vi "Test CAN write.vi"() -> ()   [LabVIEW 2023, in "PCAN API.lvlib"]
uses:
  PCAN API.lvlib
panel:
  in  "stop":bool
  out "MessageBuffer out":T1
  in  "MessageBuffer":T2(array[cluster])=[{"ID"=225, "MSGTYPE"=0, "LEN"=8, "DATA[0]"=0, "DATA[1]"=6, "DATA[2]"=0, "DATA[3]"=6, "DATA[4]"=0, "DATA[5]"=6, "DATA[6]"=0, "DATA[7]"=0}, {"ID"=225, "MSGTYPE"=0, "LEN"=8, "DATA[0]"=0, "DATA[1]"=0, "DATA[2]"=6, "DATA[3]"=2, "DATA[4]"=0, "DATA[5]"=5, "DATA[6]"=0, "DATA[7]"=0}, {"ID"=225, "MSGTYPE"=0, "LEN"=8, "DATA[0]"=8, "DATA[1]"=0, "DATA[2]"=0, "DATA[3]"=7, "DATA[4]"=0, "DATA[5]"=0, "DATA[6]"=0, "DATA[7]"=0}, {"ID"=225, "MSGTYPE"=0, "LEN"=8, "DATA[0]"=0, "DATA[1]"=0, "DATA[2]"=5, "DATA[3]"=0, "DATA[4]"=0, "DATA[5]"=0, "DATA[6]"=6, "DATA[7]"=0}, {"ID"=225, "MSGTYPE"=0, "LEN"=8, "DATA[0]"=0, "DATA[1]"=0, "DATA[2]"=7, "DATA[3]"=8, "DATA[4]"=8, "DATA[5]"=0, "DATA[6]"=0, "DATA[7]"=0}, {"ID"=225, "MSGTYPE"=0, "LEN"=8, "DATA[0]"=0, "DATA[1]"=3, "DATA[2]"=4, "DATA[3]"=6, "DATA[4]"=0, "DATA[5]"=0, "DATA[6]"=0, "DATA[7]"=0}, {"ID"=225, "MSGTYPE"=0, "LEN"=8, "DATA[0]"=1, "DATA[1]"=1, "DATA[2]"=1, "DATA[3]"=1, "DATA[4]"=0, "DATA[5]"=0, "DATA[6]"=0, "DATA[7]"=0}] {"ID" format="%.0x"}
  out "error out 2":errorcluster
  out "error out":errorcluster
  in  "error in":errorcluster
  in  "Channel":u16=81 format="%x"
  in  "IOPort":u32 format="%x"
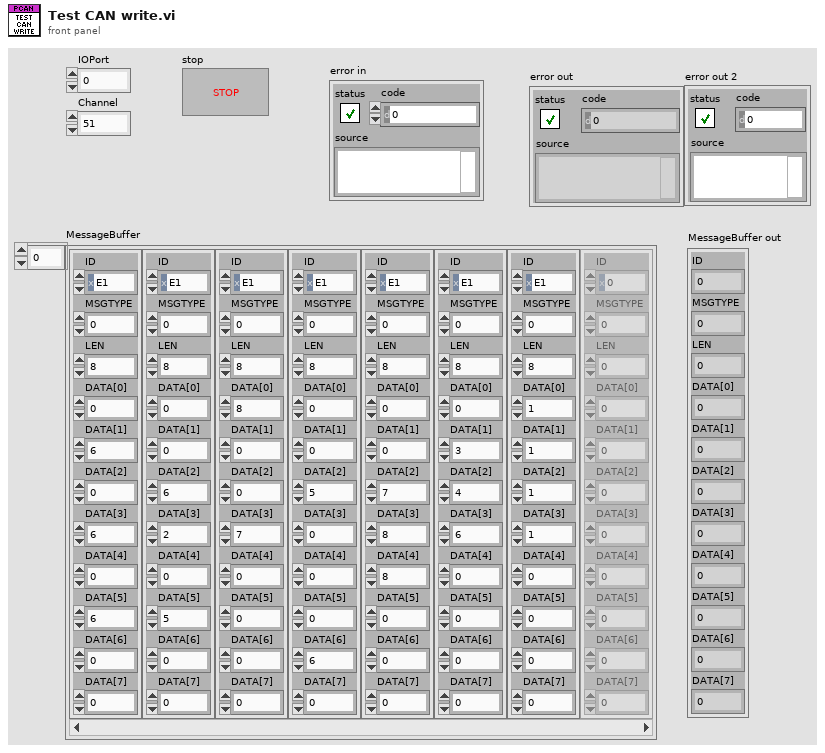
[diagram p1: front panel]
types:
  T1 = cluster{"ID":u32, "MSGTYPE":u8, "LEN":u8, "DATA[0]":u8, "DATA[1]":u8, "DATA[2]":u8, "DATA[3]":u8, "DATA[4]":u8, "DATA[5]":u8, "DATA[6]":u8, "DATA[7]":u8}
  T2 = cluster{"ID":u32, "MSGTYPE":u8, "LEN":u8, "DATA[0]":u8, "DATA[1]":u8, "DATA[2]":u8, "DATA[3]":u8, "DATA[4]":u8, "DATA[5]":u8, "DATA[6]":u8, "DATA[7]":u8}[]
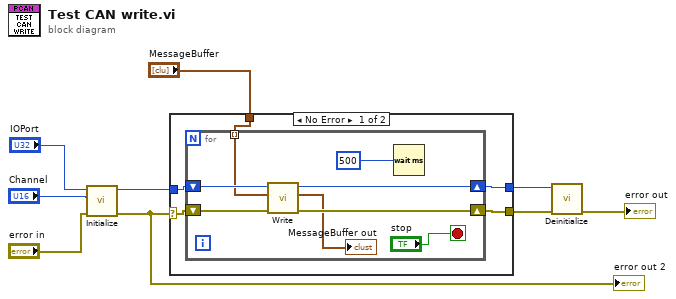
[diagram p0: block diagram]
diagram:
  n1 = call "Initialize.vi"("error in"="error in", "Channel"="Channel", "IOPort"="IOPort") -> ("error out"=w2:errorcluster, "Channel"=w6:u16)  [unwired: 6 in, 1 out]
  "error out 2" <- w2
  n2 = case shown="No Error" w2 {
    selector: w2 -> [w14 w23]
    tunnel: [w13 w23] -> w4
    tunnel: w6 -> [w12 w24]
    tunnel: [w11 w24] -> w5
    tunnel: "MessageBuffer" -> [w10 _]
    frame No Error {
      n3 = for {
        shift-right: [w21] -> w13
        shift-left: w14 -> [w22]
        shift-right: [w19] -> w11
        shift-left: w12 -> [w20]
        tunnel: w10 -> [w16] mode=indexing
        stop <- "stop" stop-if-true
        n4 = call "Write.vi"("error in"=w22, "MessageBuffer"=w16, "Channel"=w20) -> ("error out"=w21:errorcluster, "MessageBuffer out"=→"MessageBuffer out":T1, "Channel out"=w19:u16)  [unwired: 5 in, 1 out]
        n5 = Wait (ms)(milliseconds to wait=u32 500) -> ()  [unwired: 1 out]
      }
    }
    frame Error {
    }
  }
  n6 = call "Deinitialize.vi"("error in"=w4, "Channel"=w5) -> ("error out"=→"error out":errorcluster)  [unwired: 9 in]
